vi "IDA_REGRESO_COMPLETO_sin parametrizar.vi"() -> ()   [LabVIEW 2014]
uses:
  <vilib>/MakerHub/LINX/Public/Peripherals/Digital/Digital Read 1 Chan.vi
  <vilib>/MakerHub/LINX/Public/Peripherals/Digital/Digital Write 1 Chan.vi
  <vilib>/MakerHub/LINX/LMH-LINX.lvlib
panel:
  out "X en origen":bool
  out "Z en origen":bool
  out "FinX":dbl
  out "FinY":dbl
  out "FinZ":dbl
  out "Y en origen":bool
  out "finZ2trunc":dbl
  out "finZtrunc":dbl
  out "finYtrunc":dbl
  out "finY2trunc":dbl
  out "finX2trunc":dbl
  out "finXtrunc":dbl
  in  "mmX":dbl
  in  "mmY":dbl
  in  "mmZ":dbl
  out "sensorZR":i16
  out "sensorYR":i16
  out "sensorXR":i16
  out "Regreso":bool
  out "Ida":bool
  out "INICIO":i16
  in  "TIPO DE DESPLAZAMIENTO":enum32{"IDA", "REGRESO"}(radio)
  out "sensorXI":i16
  out "sensorYI":i16
  out "sensorZI":i16
  in  "OK Button":bool
  out "Llegada a posición X":bool
  out "Llegada a posición Y":bool
  out "Llegada a posición Z":bool
  in  "Milisegundos de retraso":u32
  in  "cmX":dbl
  in  "cmY":dbl
  in  "cmZ":dbl
  out "Sentido X":dbl
  out "Pasos del indicador":i32
  out "Motor X":dbl(knob) scale=0.0..127.0
  out "Pasos X en sentido X":i32
  out "Sentido Y":dbl
  out "Pasos del indicador":i32
  out "Motor Y":dbl(knob) scale=0.0..127.0
  out "Pasos Y en sentido":i32
  out "Sentido Z":dbl
  out "Pasos Motor X":bool[](array[boolean])
  out "Pasos Motor Y":bool[](array[boolean])
  out "Pasos del indicador":i32
  out "Motor Z":dbl(knob) scale=0.0..127.0
  out "Pasos Z en sentido":i32
  in  "stop 2":bool
  out "Pasos Motor Z":bool[](array[boolean])
  # "COORDENADAS FINALES"
  # "Centímetros"
  # "Milímetros"
  # "Pasos a recorrer"
  # "Pasos recorridos"
  # "X"
  # "Y"
  # "Z"
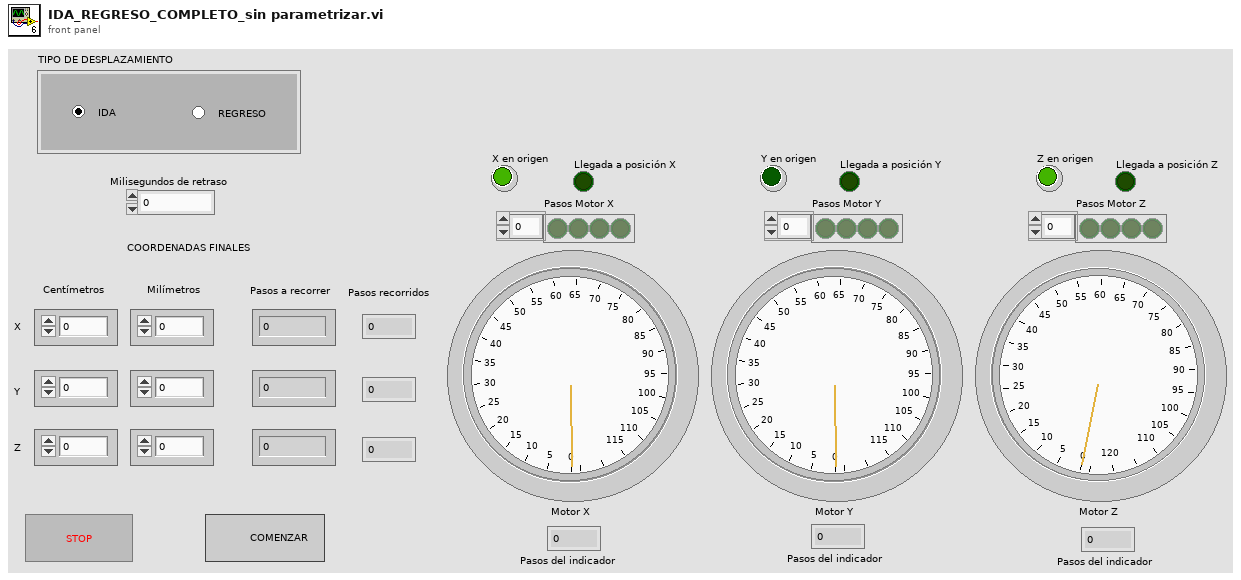
[diagram p1: front panel]
types:
  T1 = enum8{"Enabled", "Disabled", "Disabled and Grayed Out"}
  T2 = typedef "LMH-LINX.lvlib/LINX Ref.ctl" = cluster{"Platform":T3, "Interface":T4, "LINX Device Config":T5}
  T3 = typedef "LMH-LINX.lvlib/Platform.ctl" = enum16{"LINX", "myRIO"}
  T4 = typedef "LMH-LINX.lvlib/Interface.ctl" = enum16{"Serial", "TCP"}
  T5 = typedef "LMH-LINX.lvlib/Device.lvlib/LINX Device Config.ctl" = cluster{"Interface":T4, "COM Port":refnum<visa-resource-name>, "TCP Configuration":T6, "Device Family":u8, "Device ID":u8, "Device Name":string, "TCP Ref":refnum<k5>, "Channels":T7}
  T6 = typedef "LMH-LINX.lvlib/Device.lvlib/TCP Config.ctl" = cluster{"IP Address":string, "Port":u16}
  T7 = typedef "LMH-LINX.lvlib/Channels.ctl" = cluster{"DI":u8[], "DO":u8[], "AI":u8[], "AO":u8[], "PWM":u8[], "QE":u8[], "UART":u8[], "I2C 2":u8[], "SPI":u8[], "CAN":u8[], "Servo":u8[], "AI Ref (V)":dbl, "AO Ref (V)":dbl, "AO Resolution (Bits)":u8}
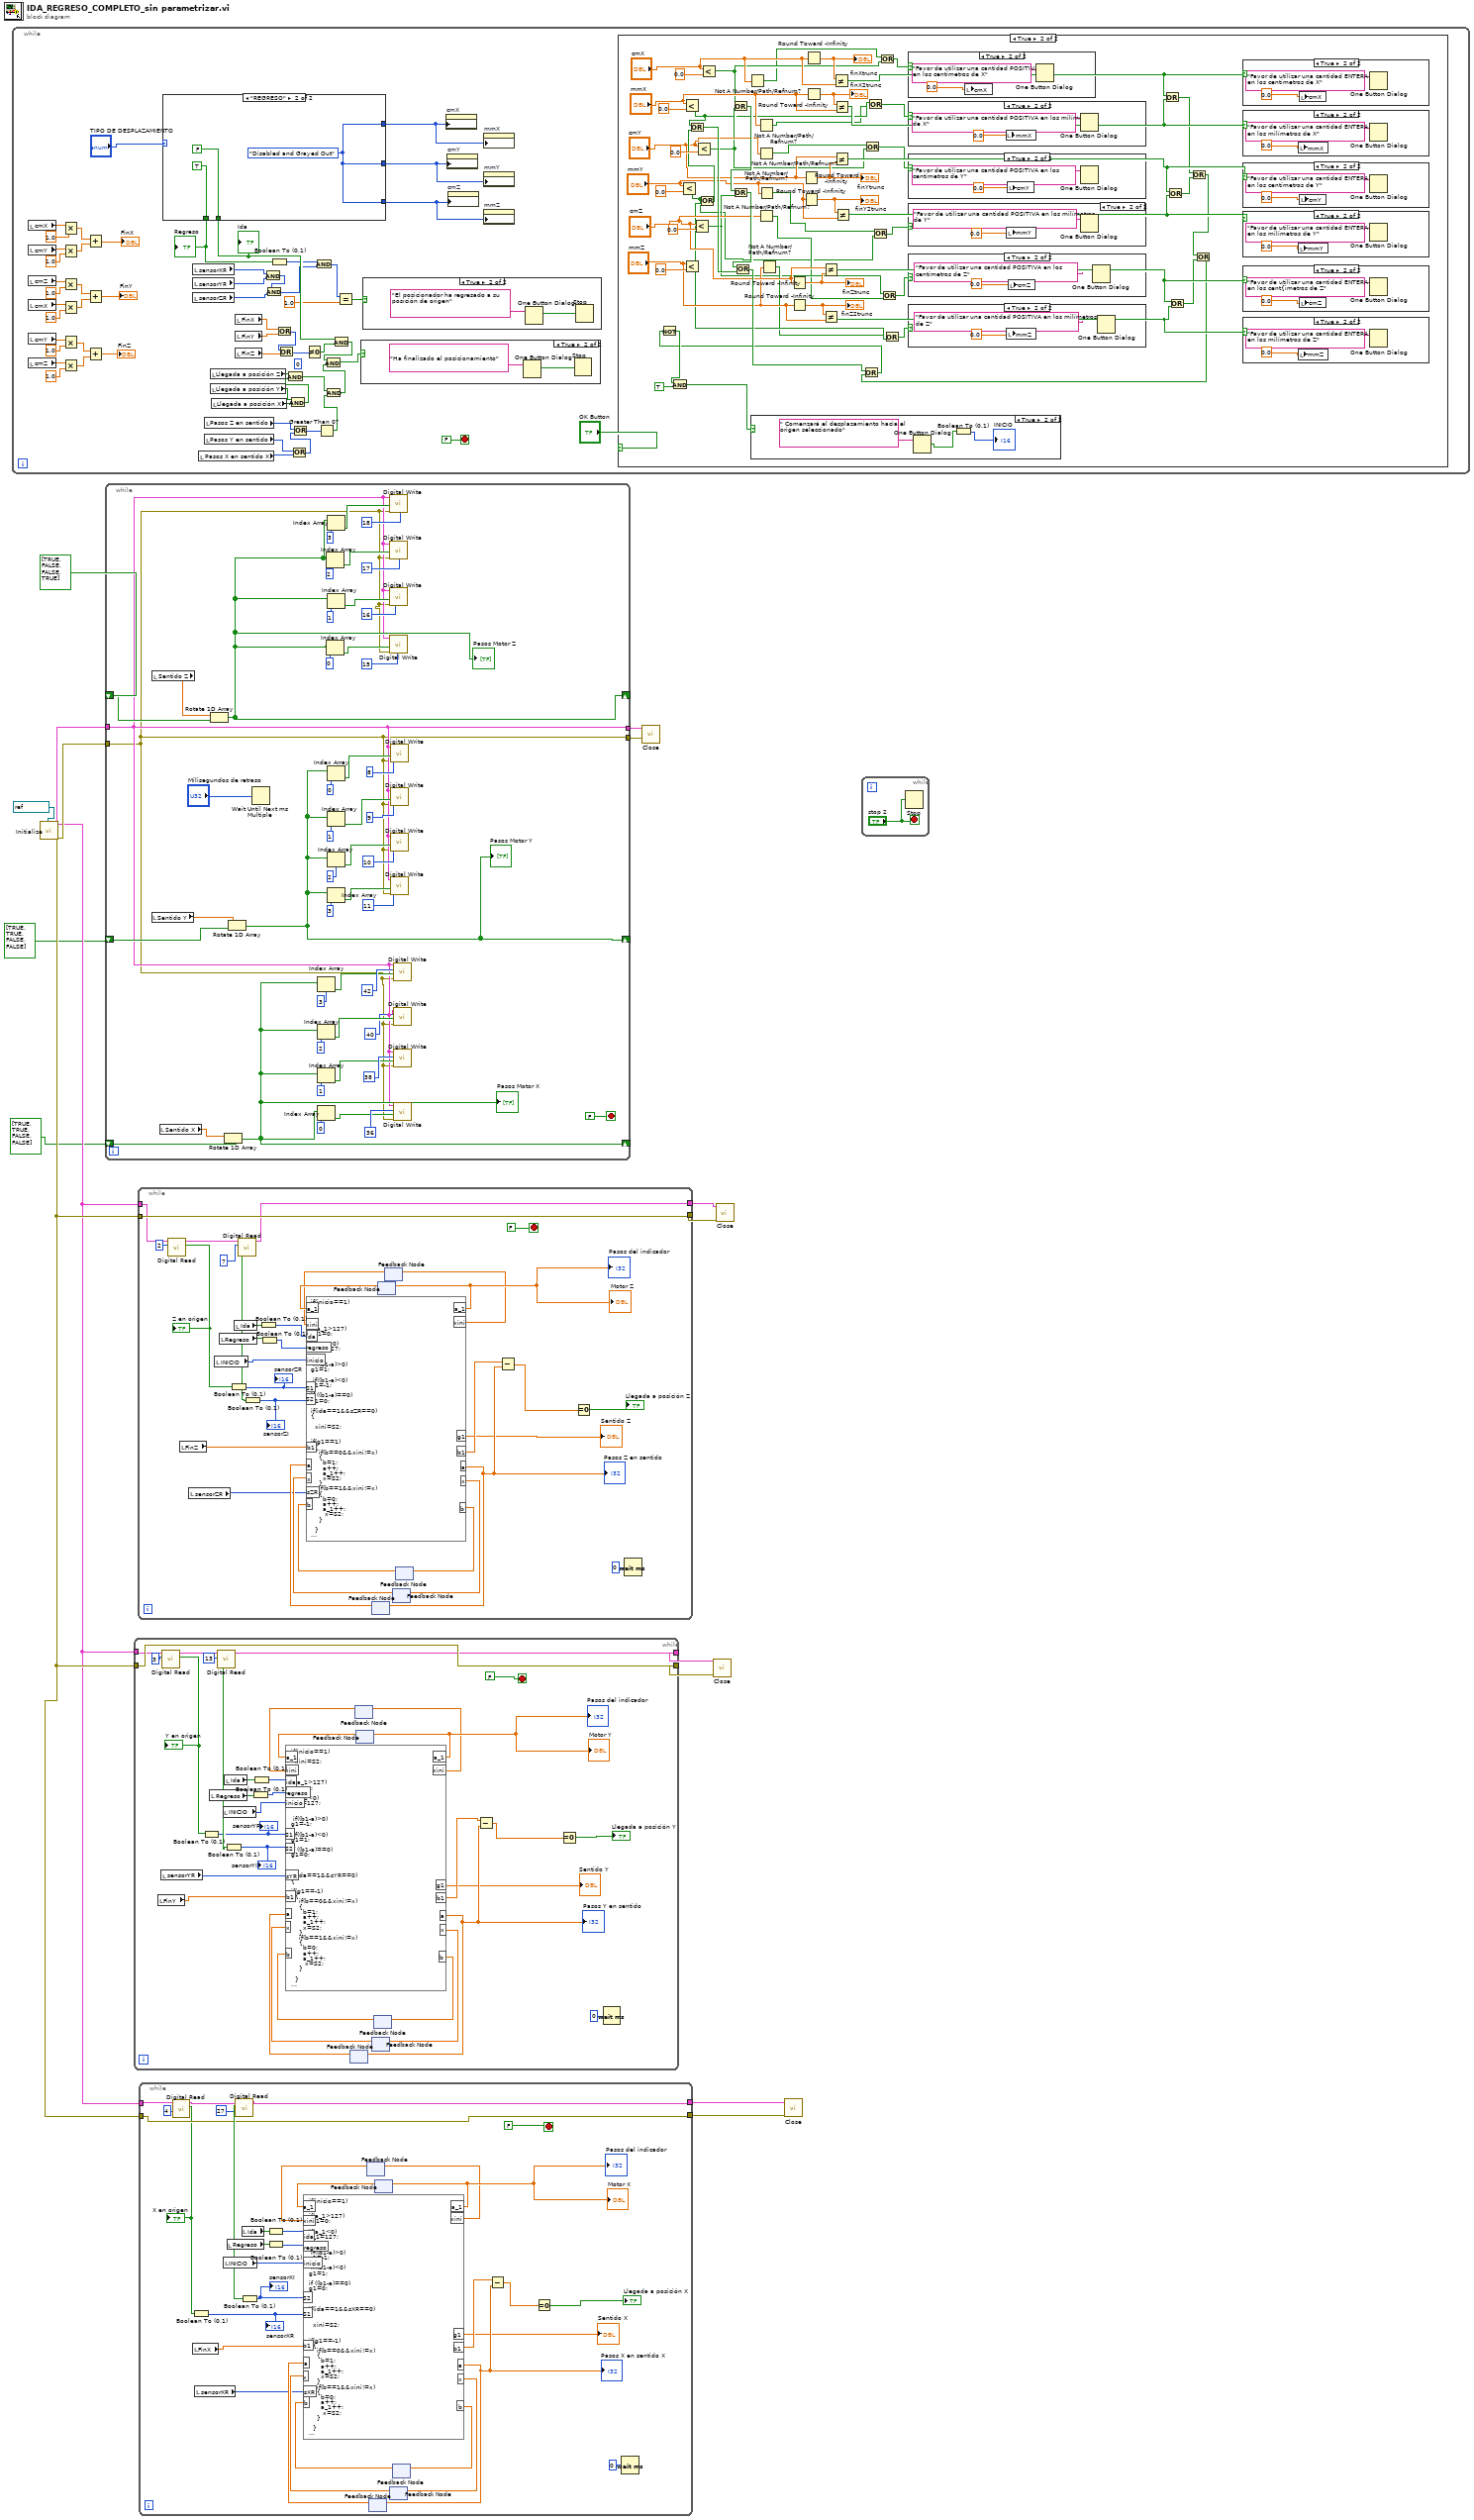
[diagram p0: block diagram]
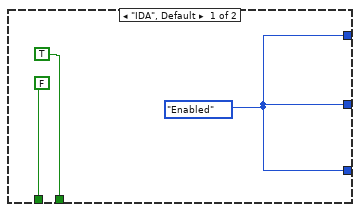
[diagram p4: hidden frame]
diagram:
  n1 = while {
    stop <- FALSE stop-if-true
    (unwired) 0 ("y")
    n2 = local read "cmX"() -> (w37:dbl)
    n3 = local read "cmY"() -> (w36:dbl)
    n4 = local read "cmZ"() -> (w35:dbl)
    n5 = local read "cmX"() -> (w34:dbl)
    n6 = local read "cmY"() -> (w33:dbl)
    n7 = local read "cmZ"() -> (w38:dbl)
    n8 = Multiply(x=w37, y=1.0) -> (x*y=w23:dbl)
    n9 = Multiply(x=w36, y=1.0) -> (x*y=w26:dbl)
    n10 = Multiply(x=w35, y=1.0) -> (x*y=w22:dbl)
    n11 = Multiply(x=w34, y=1.0) -> (x*y=w25:dbl)
    n12 = Multiply(x=w33, y=1.0) -> (x*y=w21:dbl)
    n13 = Multiply(x=w38, y=1.0) -> (x*y=w24:dbl)
    n14 = Add(x=w23, y=w26) -> (x+y=→"FinX":dbl)
    n15 = Add(x=w22, y=w25) -> (x+y=→"FinY":dbl)
    n16 = Add(x=w21, y=w24) -> (x+y=→"FinZ":dbl)
    n17 = case shown="\"REGRESO\"" "TIPO DE DESPLAZAMIENTO" {
      tunnel: [w79 w82] -> w15
      tunnel: [w79 w82] -> w16
      tunnel: [w79 w82] -> w17
      tunnel: [TRUE FALSE] -> w50
      tunnel: [FALSE TRUE] -> w42
      frame "IDA", Default {
        w79 = T1."Enabled" ("Disabled")
      }
      frame "REGRESO" {
        w82 = T1."Disabled and Grayed Out" ("Disabled")
      }
    }
    "Ida" <- w50
    "Regreso" <- w42
    n18 = local read "sensorXR"() -> (w48:i16)
    n19 = local read "sensorYR"() -> (w47:i16)
    n20 = local read "sensorZR"() -> (w46:i16)
    n21 = local read "Pasos X en sentido X"() -> (w57:i32)
    n22 = local read "Pasos Z en sentido"() -> (w56:i32)
    n23 = local read "Pasos Y en sentido"() -> (w58:i32)
    n24 = local read "Llegada a posición Z"() -> (w67:bool)
    n25 = local read "Llegada a posición Y"() -> (w66:bool)
    n26 = local read "Llegada a posición X"() -> (w65:bool)
    n27 = local read "FinX"() -> (w62:dbl)
    n28 = local read "FinY"() -> (w63:dbl)
    n29 = local read "FinZ"() -> (w64:dbl)
    n30 = And(x=w48, y=w47) -> (x .and. y?=w45:i16)
    n31 = And(x=w45, y=w46) -> (x .and. y?=w40:i16)
    n32 = Boolean To (0,1)(Boolean=w42) -> (0, 1=w41:i16)
    n33 = Or(x=w62, y=w63) -> (x .or. y?=w61:i32)
    n34 = Or(x=w61, y=w64) -> (x .or. y?=w60:i32)
    n35 = And(x=w66, y=w65) -> (x .and. y?=w69:bool)
    n36 = And(x=w67, y=w69) -> (x .and. y?=w55:bool)
    n37 = Or(x=w58, y=w57) -> (x .or. y?=w59:i32)
    n38 = Or(x=w56, y=w59) -> (x .or. y?=w54:i32)
    n39 = Not Equal To 0?(x=w60) -> (x != 0?=w49:bool)
    n40 = And(x=w41, y=w40) -> (x .and. y?=w39:i16)
    n41 = Greater Than 0?(x=w54) -> (x > 0?=w53:bool)
    n42 = And(x=w55, y=w53) -> (x .and. y?=w52:bool)
    n43 = And(x=w50, y=w49) -> (x .and. y?=w51:bool)
    n44 = And(x=w51, y=w52) -> (x .and. y?=w68:bool)
    n45 = Equal?(x=w39, y=1.0) -> (x = y?=w43:bool)
    n46 = case shown="True" w68 {
      frame False {
      }
      frame True {
        n47 = One Button Dialog(message="Ha finalizado el posicionamiento") -> (true=w75:bool)  [unwired: 1 in]
        n48 = Stop(stop? (T)=w75) -> ()
      }
    }
    n49 = case shown="True" w43 {
      frame False {
      }
      frame True {
        n50 = One Button Dialog(message="El posicionador ha regresado a su posición de origen") -> (true=w73:bool)  [unwired: 1 in]
        n51 = Stop(stop? (T)=w73) -> ()
      }
    }
    n52 = property on="cmX" class="DigNum (strict)"("DisabledEnum"=w17) -> ()  [unwired: 2 in, 2 out]
    n53 = property on="cmY" class="DigNum (strict)"("DisabledEnum"=w16) -> ()  [unwired: 2 in, 2 out]
    n54 = property on="cmZ" class="DigNum (strict)"("DisabledEnum"=w15) -> ()  [unwired: 2 in, 2 out]
    n55 = property on="mmX" class="DigNum (strict)"("DisabledEnum"=w17) -> ()  [unwired: 2 in, 2 out]
    n56 = property on="mmY" class="DigNum (strict)"("DisabledEnum"=w16) -> ()  [unwired: 2 in, 2 out]
    n57 = property on="mmZ" class="DigNum (strict)"("DisabledEnum"=w15) -> ()  [unwired: 2 in, 2 out]
    n58 = case shown="True" "OK Button" {
      frame False {
      }
      frame True {
        n59 = Less?(x="mmY", y=0.0) -> (x < y?=w94:bool)
        n60 = Less?(x="mmX", y=0.0) -> (x < y?=w85:bool)
        n61 = Less?(x="mmZ", y=0.0) -> (x < y?=w100:bool)
        n62 = Less?(x="cmZ", y=0.0) -> (x < y?=w97:bool)
        n63 = Less?(x="cmY", y=0.0) -> (x < y?=w91:bool)
        n64 = Or(x=w94, y=w100) -> (x .or. y?=w129:bool)
        n65 = Or(x=w85, y=w129) -> (x .or. y?=w127:bool)
        n66 = Less?(x="cmX", y=0.0) -> (x < y?=w88:bool)
        n67 = Or(x=w88, y=w91) -> (x .or. y?=w133:bool)
        n68 = Or(x=w133, y=w97) -> (x .or. y?=w128:bool)
        n69 = Or(x=w128, y=w127) -> (x .or. y?=w109:bool)
        n70 = Not A Number/Path/Refnum?(number/path/refnum="cmX") -> (NaN/Path/Refnum?=w87:bool)
        n71 = Not A Number/Path/Refnum?(number/path/refnum="mmX") -> (NaN/Path/Refnum?=w83:bool)
        n72 = Not A Number/Path/Refnum?(number/path/refnum="cmY") -> (NaN/Path/Refnum?=w89:bool)
        n73 = Not A Number/Path/Refnum?(number/path/refnum="cmZ") -> (NaN/Path/Refnum?=w95:bool)
        n74 = Not A Number/Path/Refnum?(number/path/refnum="mmY") -> (NaN/Path/Refnum?=w92:bool)
        n75 = Not A Number/Path/Refnum?(number/path/refnum="mmZ") -> (NaN/Path/Refnum?=w98:bool)
        n76 = Round Toward -Infinity(1:"cmZ") -> (0:w121:dbl)
        "finZtrunc" <- w121
        n77 = Round Toward -Infinity(1:"mmZ") -> (0:w120:dbl)
        "finZ2trunc" <- w120
        n78 = Round Toward -Infinity(1:"cmY") -> (0:w123:dbl)
        "finYtrunc" <- w123
        n79 = Round Toward -Infinity(1:"mmY") -> (0:w122:dbl)
        "finY2trunc" <- w122
        n80 = Round Toward -Infinity(1:"cmX") -> (0:w126:dbl)
        "finXtrunc" <- w126
        n81 = Round Toward -Infinity(1:"mmX") -> (0:w125:dbl)
        "finX2trunc" <- w125
        n82 = Not Equal?(x="cmZ", y=w121) -> (x != y?=w115:bool)
        n83 = Not Equal?(x=w120, y="mmZ") -> (x != y?=w114:bool)
        n84 = Not Equal?(x=w126, y="cmX") -> (x != y?=w119:bool)
        n85 = Not Equal?(x=w125, y="mmX") -> (x != y?=w118:bool)
        n86 = Not Equal?(x="cmY", y=w123) -> (x != y?=w117:bool)
        n87 = Not Equal?(x=w122, y="mmY") -> (x != y?=w116:bool)
        n88 = Or(x=w89, y=w91) -> (x .or. y?=w90:bool)
        n89 = Or(x=w85, y=w83) -> (x .or. y?=w84:bool)
        n90 = Or(x=w92, y=w94) -> (x .or. y?=w93:bool)
        n91 = Or(x=w87, y=w88) -> (x .or. y?=w86:bool)
        n92 = Or(x=w97, y=w95) -> (x .or. y?=w96:bool)
        n93 = Or(x=w98, y=w100) -> (x .or. y?=w99:bool)
        n94 = case shown="True" w86 {
          frame False {
          }
          frame True {
            n95 = local write "cmX"(0.0 ("IniX")) -> ()
            n96 = One Button Dialog(message="Favor de utilizar una cantidad POSITIVA en los centímetros de X") -> ()  [unwired: 1 in, 1 out]
          }
        }
        n97 = case shown="True" w84 {
          frame False {
          }
          frame True {
            n98 = local write "mmX"(0.0 ("IniY")) -> ()
            n99 = One Button Dialog(message="Favor de utilizar una cantidad POSITIVA en los milímetros de X") -> ()  [unwired: 1 in, 1 out]
          }
        }
        n100 = case shown="True" w90 {
          frame False {
          }
          frame True {
            n101 = local write "cmY"(0.0 ("IniY")) -> ()
            n102 = One Button Dialog(message="Favor de utilizar una cantidad POSITIVA en los centímetros de Y") -> ()  [unwired: 1 in, 1 out]
          }
        }
        n103 = case shown="True" w93 {
          frame False {
          }
          frame True {
            n104 = local write "mmY"(0.0 ("IniZ")) -> ()
            n105 = One Button Dialog(message="Favor de utilizar una cantidad POSITIVA en los milímetros de Y") -> ()  [unwired: 1 in, 1 out]
          }
        }
        n106 = case shown="True" w96 {
          frame False {
          }
          frame True {
            n107 = local write "cmZ"(0.0 ("IniZ")) -> ()
            n108 = One Button Dialog(message="Favor de utilizar una cantidad POSITIVA en los centímetros de Z") -> ()  [unwired: 1 in, 1 out]
          }
        }
        n109 = case shown="True" w99 {
          frame False {
          }
          frame True {
            n110 = local write "mmZ"(0.0 ("IniZ")) -> ()
            n111 = One Button Dialog(message="Favor de utilizar una cantidad POSITIVA en los milímetros de Z") -> ()  [unwired: 1 in, 1 out]
          }
        }
        n112 = Or(x=w119, y=w118) -> (x .or. y?=w113:bool)
        n113 = Or(x=w117, y=w116) -> (x .or. y?=w112:bool)
        n114 = Or(x=w115, y=w114) -> (x .or. y?=w110:bool)
        n115 = Or(x=w113, y=w112) -> (x .or. y?=w111:bool)
        n116 = Or(x=w111, y=w110) -> (x .or. y?=w108:bool)
        n117 = Or(x=w109, y=w108) -> (x .or. y?=w107:bool)
        n118 = Not(x=w107) -> (.not. x?=w132:bool)
        n119 = And(x=w132, y=TRUE) -> (x .and. y?=w135:bool)
        n120 = case shown="True" w135 {
          frame False {
          }
          frame True {
            n121 = One Button Dialog(message=" Comenzará el desplazamiento hacia el origen seleccionado") -> (true=w158:bool)  [unwired: 1 in]
            n122 = Boolean To (0,1)(Boolean=w158) -> (0, 1=→"INICIO":i16)
          }
        }
        n123 = case shown="True" w119 {
          frame False {
          }
          frame True {
            n124 = local write "cmX"(0.0 ("IniX")) -> ()
            n125 = One Button Dialog(message="Favor de utilizar una cantidad ENTERA en los centímetros de X") -> ()  [unwired: 1 in, 1 out]
          }
        }
        n126 = case shown="True" w118 {
          frame False {
          }
          frame True {
            n127 = local write "mmX"(0.0 ("IniX")) -> ()
            n128 = One Button Dialog(message="Favor de utilizar una cantidad ENTERA en los milímetros de X") -> ()  [unwired: 1 in, 1 out]
          }
        }
        n129 = case shown="True" w117 {
          frame False {
          }
          frame True {
            n130 = local write "cmY"(0.0 ("IniX")) -> ()
            n131 = One Button Dialog(message="Favor de utilizar una cantidad ENTERA en los centímetros de Y") -> ()  [unwired: 1 in, 1 out]
          }
        }
        n132 = case shown="True" w116 {
          frame False {
          }
          frame True {
            n133 = local write "mmY"(0.0 ("IniX")) -> ()
            n134 = One Button Dialog(message="Favor de utilizar una cantidad ENTERA en los milímetros de Y") -> ()  [unwired: 1 in, 1 out]
          }
        }
        n135 = case shown="True" w115 {
          frame False {
          }
          frame True {
            n136 = local write "cmZ"(0.0 ("IniX")) -> ()
            n137 = One Button Dialog(message="Favor de utilizar una cantidad ENTERA en los cent{imetros de Z") -> ()  [unwired: 1 in, 1 out]
          }
        }
        n138 = case shown="True" w114 {
          frame False {
          }
          frame True {
            n139 = local write "mmZ"(0.0 ("IniX")) -> ()
            n140 = One Button Dialog(message="Favor de utilizar una cantidad ENTERA en los milímetros de Z") -> ()  [unwired: 1 in, 1 out]
          }
        }
      }
    }
  }
  n141 = call <vilib>:"Initialize.vi"("Serial Port"=refnum<visa-resource-name> "COM4") -> ("Error Out"=w10:errorcluster, "LINX Ref"=w9:T2)  [unwired: 8 in, 1 out]
  n142 = while {
    shift-right: [w168] -> _
    shift-left: bool[] [TRUE, FALSE, FALSE, TRUE] -> [w210]
    tunnel: w9 -> [w167]
    tunnel: w10 -> [w166]
    shift-right: [w169] -> _
    shift-left: bool[] [TRUE, TRUE, FALSE, FALSE] -> [w185]
    shift-right: [w170] -> _
    shift-left: bool[] [TRUE, TRUE, FALSE, FALSE] -> [w171]
    tunnel: [w167] -> w4
    tunnel: [w166] -> w3
    stop <- FALSE stop-if-true
    n143 = local read "Sentido Y"() -> (w198:dbl)
    n144 = local read "Sentido Z"() -> (w200:dbl)
    n145 = local read "Sentido X"() -> (w172:dbl)
    n146 = Rotate 1D Array(1:w210, 2:w200) -> (0:w168:bool[])
    "Pasos Motor Z" <- w168
    n147 = Rotate 1D Array(1:w171, 2:w172) -> (0:w170:bool[])
    "Pasos Motor X" <- w170
    n148 = Rotate 1D Array(1:w185, 2:w198) -> (0:w169:bool[])
    "Pasos Motor Y" <- w169
    n149 = Wait Until Next ms Multiple(millisecond multiple="Milisegundos de retraso") -> ()  [unwired: 1 out]
    n150 = Index Array(array=w170, index=3) -> (element=w173:bool)
    n151 = Index Array(array=w170, index=2) -> (element=w176:bool)
    n152 = Index Array(array=w170, index=1) -> (element=w177:bool)
    n153 = Index Array(array=w170, index=0) -> (element=w179:bool)
    n154 = Index Array(array=w168, index=2) -> (element=w205:bool)
    n155 = Index Array(array=w168, index=0) -> (element=w208:bool)
    n156 = Index Array(array=w168, index=3) -> (element=w202:bool)
    n157 = Index Array(array=w168, index=1) -> (element=w206:bool)
    n158 = Index Array(array=w169, index=0) -> (element=w191:bool)
    n159 = Index Array(array=w169, index=1) -> (element=w193:bool)
    n160 = Index Array(array=w169, index=2) -> (element=w194:bool)
    n161 = Index Array(array=w169, index=3) -> (element=w197:bool)
    n162 = call-poly <vilib>:"Digital Write.vi"("Error In"=w166, "Output Value"=w202, "DO Channel"=u8 18 ("Digital I/O Pin (0)"), "LINX Resource"=w167) -> ()  [unwired: 6 in, 2 out]
    n163 = call-poly <vilib>:"Digital Write.vi"("Error In"=w166, "Output Value"=w205, "DO Channel"=u8 17 ("Digital I/O Pin (0)"), "LINX Resource"=w167) -> ()  [unwired: 6 in, 2 out]
    n164 = call-poly <vilib>:"Digital Write.vi"("Error In"=w166, "Output Value"=w206, "DO Channel"=u8 16 ("Digital I/O Pin (0)"), "LINX Resource"=w167) -> ()  [unwired: 6 in, 2 out]
    n165 = call-poly <vilib>:"Digital Write.vi"("Error In"=w166, "Output Value"=w208, "DO Channel"=u8 15 ("Digital I/O Pin (0)"), "LINX Resource"=w167) -> ()  [unwired: 6 in, 2 out]
    n166 = call-poly <vilib>:"Digital Write.vi"("Error In"=w166, "Output Value"=w191, "DO Channel"=u8 8 ("Digital I/O Pin (0)"), "LINX Resource"=w167) -> ()  [unwired: 6 in, 2 out]
    n167 = call-poly <vilib>:"Digital Write.vi"("Error In"=w166, "Output Value"=w193, "DO Channel"=u8 9 ("Digital I/O Pin (0)"), "LINX Resource"=w167) -> ()  [unwired: 6 in, 2 out]
    n168 = call-poly <vilib>:"Digital Write.vi"("Error In"=w166, "Output Value"=w194, "DO Channel"=u8 10 ("Digital I/O Pin (0)"), "LINX Resource"=w167) -> ()  [unwired: 6 in, 2 out]
    n169 = call-poly <vilib>:"Digital Write.vi"("Error In"=w166, "Output Value"=w197, "DO Channel"=u8 11 ("Digital I/O Pin (0)"), "LINX Resource"=w167) -> ()  [unwired: 6 in, 2 out]
    n170 = call-poly <vilib>:"Digital Write.vi"("Error In"=w166, "Output Value"=w173, "DO Channel"=u8 42 ("Digital I/O Pin (0)"), "LINX Resource"=w167) -> ()  [unwired: 6 in, 2 out]
    n171 = call-poly <vilib>:"Digital Write.vi"("Error In"=w166, "Output Value"=w176, "DO Channel"=u8 40 ("Digital I/O Pin (0)"), "LINX Resource"=w167) -> ()  [unwired: 6 in, 2 out]
    n172 = call-poly <vilib>:"Digital Write.vi"("Error In"=w166, "Output Value"=w177, "DO Channel"=u8 38 ("Digital I/O Pin (0)"), "LINX Resource"=w167) -> ()  [unwired: 6 in, 2 out]
    n173 = call-poly <vilib>:"Digital Write.vi"("Error In"=w166, "Output Value"=w179, "DO Channel"=u8 36 ("Digital I/O Pin (0)"), "LINX Resource"=w167) -> ()  [unwired: 6 in, 2 out]
  }
  n174 = while {
    tunnel: w10 -> [w236]
    tunnel: w9 -> [w220]
    tunnel: [w235] -> w12
    tunnel: [w236] -> w7
    stop <- FALSE stop-if-true
    n175 = local read "FinY"() -> (w215:dbl)
    n176 = local read "sensorYR"() -> (w216:i16)
    n177 = call-poly <vilib>:"Digital Read.vi"("DI Channel"=u8 3, "LINX Resource"=w220) -> ("DI Value"=w217:bool, "LINX Resource"=w221:T2)  [unwired: 7 in, 1 out]
    "Y en origen" <- w217
    n178 = Boolean To (0,1)(Boolean=w217) -> (0, 1=w218:i16)
    "sensorYR" <- w218
    n179 = local read "Regreso"() -> (w224:bool)
    n180 = call-poly <vilib>:"Digital Read.vi"("DI Channel"=u8 13, "LINX Resource"=w221) -> ("DI Value"=w247:bool, "LINX Resource"=w235:T2)  [unwired: 7 in, 1 out]
    n181 = local read "INICIO"() -> (w227:i16)
    n182 = local read "Ida"() -> (w225:bool)
    n183 = Boolean To (0,1)(Boolean=w247) -> (0, 1=w246:i16)
    "sensorYI" <- w246
    n184 = Boolean To (0,1)(Boolean=w224) -> (0, 1=w222:i16)
    n185 = Boolean To (0,1)(Boolean=w225) -> (0, 1=w223:i16)
    n186 = feedback #1() -> (w239:dbl)  [unwired: 1 in]
    n187 = feedback #2() -> (w229:dbl)  [unwired: 1 in]
    n188 = feedback #3() -> (w244:dbl)  [unwired: 1 in]
    n189 = feedback #4() -> (w242:dbl)  [unwired: 1 in]
    n190 = feedback #5() -> (w241:dbl)  [unwired: 1 in]
    n191 = formula code="if(inicio==1)\n{\n  xini=S2;\n\n\n\nif(a_1>127)\na_1=0;\n\nif(a_1<0)\na_1=127;\n\n\n if((b1-a)>0)\ng1=-1;\n\n if((b1-a)<0)\ng1=1;\n\nif ((b1-a)==0)\ng1=0;\n \n\n   \nif(ida==1&&sYR==0)\n{\n\nif(g1==-1)\n  {\n    if(b==0&&xini!=x)\n    {\n      b=1;\n      a++;\n      a_1++;\n      x=S2;\n    }\n    if(b==1&&xini!=x)\n    {\n      b=0;\n      a++;\n      a_1++;\n       x=S2;\n    }\n     \n  }\n  \n  if(g1==1)\n  {\n    if(b==0&&xini!=x)\n    {\n      b=1;\n      a--;\n      a_1--;\n      x=S2;\n    }\n\n\n    if(b==1&&xini!=x)\n    {\n      b=0;\n      a--;\n      a_1--;\n      x=S2;\n    }\n  }\n}\n\n\nif(regreso==1)\n{\nif(S1==0)\n{\ng1=1;\n}\nelse\n{\ng1=0;\n}\n}\n\n\n\n\n}"("S2"=w246, "a_1"=w244, "x"=w242, "b"=w241, "a"=w239, "b1"=w215, "xini"=w229, "inicio"=w227, "ida"=w223, "regreso"=w222, "S1"=w218, "sYR"=w216) -> ("a_1"=w238:dbl, "b"=w232:dbl, "x"=w243:dbl, "a"=w233:dbl, "g1"=→"Sentido Y":dbl, "b1"=w234:dbl, "xini"=w230:dbl)
    "Pasos Y en sentido" <- w233
    "Motor Y" <- w238
    "Pasos del indicador" <- w238
    n192 = feedback-in #1(w233) -> ()
    n193 = feedback-in #2(w230) -> ()
    n194 = feedback-in #3(w238) -> ()
    n195 = feedback-in #4(w243) -> ()
    n196 = feedback-in #5(w232) -> ()
    n197 = Subtract(x=w234, y=w233) -> (x-y=w226:dbl)
    n198 = Equal To 0?(x=w226) -> (x = 0?=→"Llegada a posición Y":bool)
    n199 = Wait (ms)(milliseconds to wait=u32 0) -> ()  [unwired: 1 out]
  }
  n200 = while {
    tunnel: w10 -> [w269]
    tunnel: w9 -> [w253]
    tunnel: [w268] -> w2
    tunnel: [w269] -> w1
    stop <- FALSE stop-if-true
    n201 = call-poly <vilib>:"Digital Read.vi"("DI Channel"=u8 2, "LINX Resource"=w253) -> ("DI Value"=w250:bool, "LINX Resource"=w254:T2)  [unwired: 7 in, 1 out]
    "Z en origen" <- w250
    n202 = local read "FinZ"() -> (w248:dbl)
    n203 = local read "sensorZR"() -> (w249:i16)
    n204 = local read "INICIO"() -> (w260:i16)
    n205 = local read "Regreso"() -> (w257:bool)
    n206 = Boolean To (0,1)(Boolean=w250) -> (0, 1=w251:i16)
    "sensorZR" <- w251
    n207 = local read "Ida"() -> (w258:bool)
    n208 = call-poly <vilib>:"Digital Read.vi"("DI Channel"=u8 7, "LINX Resource"=w254) -> ("DI Value"=w280:bool, "LINX Resource"=w268:T2)  [unwired: 7 in, 1 out]
    n209 = Boolean To (0,1)(Boolean=w280) -> (0, 1=w279:i16)
    "sensorZI" <- w279
    n210 = Boolean To (0,1)(Boolean=w258) -> (0, 1=w256:i16)
    n211 = Boolean To (0,1)(Boolean=w257) -> (0, 1=w255:i16)
    n212 = feedback #6() -> (w271:dbl)  [unwired: 1 in]
    n213 = feedback #7() -> (w277:dbl)  [unwired: 1 in]
    n214 = feedback #8() -> (w262:dbl)  [unwired: 1 in]
    n215 = feedback #9() -> (w275:dbl)  [unwired: 1 in]
    n216 = feedback #10() -> (w274:dbl)  [unwired: 1 in]
    n217 = formula code="if(inicio==1)\n{\n\n\n\nif(a_1>127)\na_1=0;\n\nif(a_1<0)\na_1=127;\n\n\n if((b1-a)>0)\ng1=1;\n\n if((b1-a)<0)\ng1=-1;\n\nif ((b1-a)==0)\ng1=0;\n\nif(ida==1&&sZR==0)\n{\n\n  xini=S2;\n   \n\nif(g1==1)\n  {\n    if(b==0&&xini!=x)\n    {\n      b=1;\n      a++;\n      a_1++;\n      x=S2;\n    }\n    if(b==1&&xini!=x)\n    {\n      b=0;\n      a++;\n      a_1++;\n       x=S2;\n    }\n     \n  }\n  \n  if(g1==-1)\n  {\n    if(b==0&&xini!=x)\n    {\n      b=1;\n      a--;\n      a_1--;\n      x=S2;\n    }\n\n\n    if(b==1&&xini!=x)\n    {\n      b=0;\n      a--;\n      a_1--;\n      x=S2;\n    }\n  }\n}\n\n\n\nif(regreso==1)\n{\nif(S1==0)\n{\ng1=-1;\n}\nelse\n{\ng1=0;\n}\n}\n\n\n\n\n\n\n\n }"("S2"=w279, "a_1"=w277, "x"=w275, "b"=w274, "a"=w271, "b1"=w248, "xini"=w262, "inicio"=w260, "ida"=w256, "regreso"=w255, "S1"=w251, "sZR"=w249) -> ("a_1"=w270:dbl, "b"=w265:dbl, "x"=w276:dbl, "a"=w266:dbl, "g1"=→"Sentido Z":dbl, "b1"=w267:dbl, "xini"=w263:dbl)
    "Pasos Z en sentido" <- w266
    "Motor Z" <- w270
    "Pasos del indicador" <- w270
    n218 = feedback-in #6(w266) -> ()
    n219 = feedback-in #7(w270) -> ()
    n220 = feedback-in #8(w263) -> ()
    n221 = feedback-in #9(w276) -> ()
    n222 = feedback-in #10(w265) -> ()
    n223 = Subtract(x=w267, y=w266) -> (x-y=w259:dbl)
    n224 = Equal To 0?(x=w259) -> (x = 0?=→"Llegada a posición Z":bool)
    n225 = Wait (ms)(milliseconds to wait=u32 0) -> ()  [unwired: 1 out]
  }
  n226 = while {
    tunnel: w10 -> [w286]
    tunnel: [w302] -> w11
    tunnel: w9 -> [w287]
    tunnel: [w286] -> w8
    stop <- FALSE stop-if-true
    n227 = call-poly <vilib>:"Digital Read.vi"("DI Channel"=u8 4, "LINX Resource"=w287) -> ("DI Value"=w284:bool, "LINX Resource"=w288:T2)  [unwired: 7 in, 1 out]
    "X en origen" <- w284
    n228 = Boolean To (0,1)(Boolean=w284) -> (0, 1=w283:i16)
    "sensorXR" <- w283
    n229 = local read "FinX"() -> (w281:dbl)
    n230 = local read "sensorXR"() -> (w282:i16)
    n231 = local read "INICIO"() -> (w294:i16)
    n232 = local read "Regreso"() -> (w291:bool)
    n233 = call-poly <vilib>:"Digital Read.vi"("DI Channel"=u8 27, "LINX Resource"=w288) -> ("DI Value"=w313:bool, "LINX Resource"=w302:T2)  [unwired: 7 in, 1 out]
    n234 = Boolean To (0,1)(Boolean=w313) -> (0, 1=w312:i16)
    "sensorXI" <- w312
    n235 = local read "Ida"() -> (w292:bool)
    n236 = Boolean To (0,1)(Boolean=w292) -> (0, 1=w290:i16)
    n237 = Boolean To (0,1)(Boolean=w291) -> (0, 1=w289:i16)
    n238 = feedback #11() -> (w296:dbl)  [unwired: 1 in]
    n239 = feedback #12() -> (w305:dbl)  [unwired: 1 in]
    n240 = feedback #13() -> (w310:dbl)  [unwired: 1 in]
    n241 = feedback #14() -> (w308:dbl)  [unwired: 1 in]
    n242 = feedback #15() -> (w307:dbl)  [unwired: 1 in]
    n243 = formula code="if(inicio==1)\n{\n\nif(a_1>127)\na_1=0;\n\nif(a_1<0)\na_1=127;\n\n\n if((b1-a)>0)\ng1=-1;\n\n if((b1-a)<0)\ng1=1;\n\nif ((b1-a)==0)\ng1=0;\n\n\n\nif(ida==1&&sXR==0)\n{\n\n  xini=S2;\n   \n\nif(g1==-1)\n  {\n    if(b==0&&xini!=x)\n    {\n      b=1;\n      a++;\n      a_1++;\n      x=S2;\n    }\n    if(b==1&&xini!=x)\n    {\n      b=0;\n      a++;\n      a_1++;\n       x=S2;\n    }\n     \n  }\n  \n  if(g1==1)\n  {\n    if(b==0&&xini!=x)\n    {\n      b=1;\n      a--;\n      a_1--;\n      x=S2;\n    }\n\n\n    if(b==1&&xini!=x)\n    {\n      b=0;\n      a--;\n      a_1--;\n      x=S2;\n    }\n  }\n}\n\nif(regreso==1)\n{\nif(S1==0)\n{\ng1=1;\n}\nelse\n{\ng1=0;\n}\n}\n\n}"("S2"=w312, "a_1"=w310, "x"=w308, "b"=w307, "a"=w305, "b1"=w281, "xini"=w296, "inicio"=w294, "ida"=w290, "regreso"=w289, "S1"=w283, "sXR"=w282) -> ("a_1"=w304:dbl, "b"=w299:dbl, "x"=w309:dbl, "a"=w300:dbl, "g1"=→"Sentido X":dbl, "b1"=w301:dbl, "xini"=w297:dbl)
    "Pasos X en sentido X" <- w300
    "Motor X" <- w304
    "Pasos del indicador" <- w304
    n244 = feedback-in #11(w297) -> ()
    n245 = feedback-in #12(w300) -> ()
    n246 = feedback-in #13(w304) -> ()
    n247 = feedback-in #14(w309) -> ()
    n248 = feedback-in #15(w299) -> ()
    n249 = Subtract(x=w301, y=w300) -> (x-y=w293:dbl)
    n250 = Equal To 0?(x=w293) -> (x = 0?=→"Llegada a posición X":bool)
    n251 = Wait (ms)(milliseconds to wait=u32 0) -> ()  [unwired: 1 out]
  }
  n252 = call <vilib>:"Close.vi"("Error In"=w3, "LINX Resource"=w4) -> ()  [unwired: 8 in, 2 out]
  n253 = call <vilib>:"Close.vi"("Error In"=w7, "LINX Resource"=w12) -> ()  [unwired: 8 in, 2 out]
  n254 = call <vilib>:"Close.vi"("Error In"=w1, "LINX Resource"=w2) -> ()  [unwired: 8 in, 2 out]
  n255 = call <vilib>:"Close.vi"("Error In"=w8, "LINX Resource"=w11) -> ()  [unwired: 8 in, 2 out]
  n256 = while {
    stop <- "stop 2" stop-if-true
    n257 = Stop(stop? (T)="stop 2") -> ()
  }
